vi "Configure.vi"(8 "error in (no error)":errorcluster, 9 "Record":bool, 10 "Recording Channels":refnum<k21>="All4498", 11 "AcquireTraces in":refnum<class "AcquireTraces.lvclass">) -> (0 "error out":errorcluster, 3 "AcquireTraces out":refnum<class "AcquireTraces.lvclass">)   [LabVIEW 2014, in "AcquireTraces.lvclass"]
uses:
  AcquireTraces.lvclass
  AcquireTraces.lvclass/AcquireTraces.ctl
  <vilib>/DAQmx/configure/timing.llb/DAQmx Timing (Sample Clock).vi
  <resource>/objmgr/daqmx.rc
panel:
  out "Name":refnum<k21>
  out "error out 2":errorcluster
  out "x/y":dbl
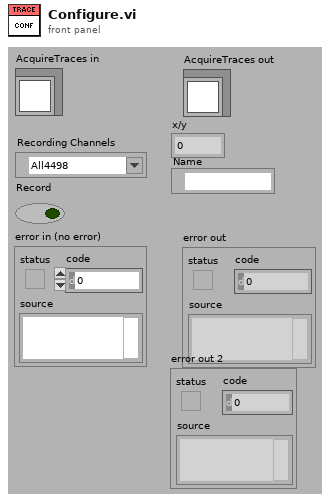
[diagram p1: front panel]
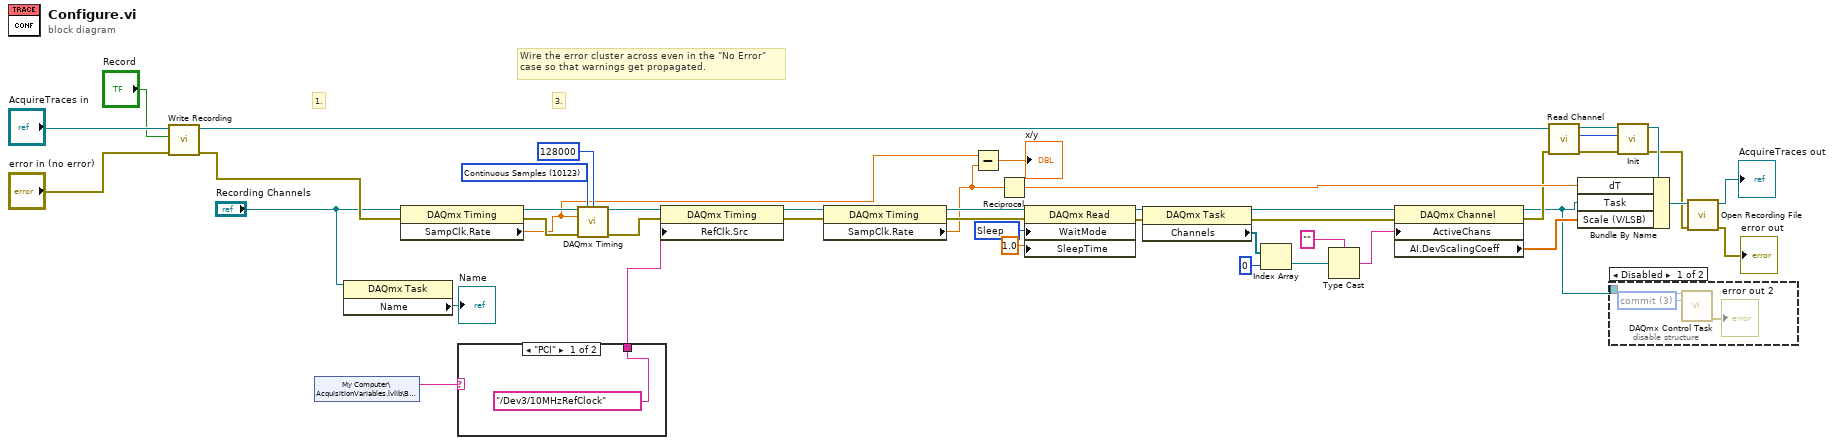
[diagram p0: block diagram]
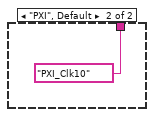
[diagram p2: hidden frame]
diagram:
  w35 = 12547 items=["Wait For Interrupt"=12523, "Poll"=12524, "Yield"=12525, "Sleep"=12547] ("WaitMode")
  w39 = 10123 items=["Finite Samples"=10178, "Continuous Samples"=10123, "Hardware Timed Single Point"=12522] ("sample mode")
  # "3."
  # "1."
  # "Wire the error cluster across even in the \"No Error\"\ncase so that warnings get propagated."
  n1 = call-dynamic "Write Recording.vi"("error in (no error)"="error in (no error)", "Recording"="Record", "AcquireTraces in"="AcquireTraces in") -> ("error out"=w9:errorcluster, "AcquireTraces out"=w6:refnum<class "AcquireTraces.lvclass">)  [unwired: 7 in]
  n2 = shared-variable "My Computer\\AcquisitionVariables.lvlib\\Bus System"() -> (w2:string)  [unwired: 1 in, 1 out]
  n3 = property class="DAQmx Task"(reference="Recording Channels") -> ("Name"=→"Name":refnum<k21>)  [unwired: 1 in, 2 out]
  n4 = property class="DAQmx Timing"(reference="Recording Channels", error in=w9) -> (reference out=w22:refnum<k21>, error out=w23:errorcluster, "SampClk.Rate"=w15:dbl)
  n5 = case shown="\"PCI\"" w2 {
    tunnel: [tag "/Dev3/10MHzRefClock" ("CI.CountEdges.Term") tag "PXI_Clk10" ("CI.CountEdges.Term")] -> w1
    frame "PCI" {
    }
    frame "PXI", Default {
    }
  }
  n6 = call-poly <vilib>:"DAQmx Timing.vi"("task/channels in"=w22, "sample mode"=w39, "samples per channel"=128000, "rate"=w15, "error in"=w23) -> ("task out"=w13:refnum<k21>, "error out"=w11:errorcluster)  [unwired: 9 in]
  n7 = property class="DAQmx Timing"(reference=w13, error in=w11, "RefClk.Src"=w1) -> (reference out=w12:refnum<k21>, error out=w10:errorcluster)
  n8 = property class="DAQmx Timing"(reference=w12, error in=w10) -> (reference out=w37:refnum<k21>, error out=w34:errorcluster, "SampClk.Rate"=w16:dbl)
  n9 = Subtract(x=w15, y=w16) -> (x-y=→"x/y":dbl)
  n10 = Reciprocal(x=w16) -> (1/x=w33:dbl)
  n11 = property class="DAQmx Read"(reference=w37, error in=w34, "WaitMode"=w35, "SleepTime"=1.0) -> (reference out=w31:refnum<k21>, error out=w30:errorcluster)
  n12 = property class="DAQmx Task"(reference=w31, error in=w30) -> (reference out=w29:refnum<k21>, error out=w28:errorcluster, "Channels"=w21:refnum<k21>[])
  n13 = Index Array(array=w21, index=0) -> (element=w26:refnum<k21>)
  n14 = Type Cast(type="", x=w26) -> (*(type *) &x=w24:string)
  n15 = property class="DAQmx Channel"(reference=w29, error in=w28, "ActiveChans"=w24) -> (reference out=w5:refnum<k21>, error out=w8:errorcluster, "AI.DevScalingCoeff"=w20:dbl[])
  n16 = call-dynamic "Read Channel.vi"("error in (no error)"=w8, "AcquistionObject in"=w6) -> ("error out"=w40:errorcluster, "Channel"=w42:i16, "AcquistionObject out"=w41:refnum<class "AcquireTraces.lvclass">)  [unwired: 7 in]
  n17 = disable-structure shown="Disabled" {
    disable-tunnel: w5 -> [w50 _]
    frame Disabled {
      w49 = 3 items=["verify"=2, "reserve"=4, "commit"=3, "unreserve"=5, "abort"=6] ("action")
      n18 = call <vilib>:"DAQmx Control Task.vi"("task/channels in"=w50, "action"=w49) -> ("error out"=→"error out 2":errorcluster)  [unwired: 12 in, 1 out]
    }
    frame Enabled {
    }
  }
  n19 = call-dynamic "Init.vi"("error in (no error)"=w40, "Channel"=w42, "AcquistionObject in"=w41) -> ("error out"=w7:errorcluster, "AcquistionObject out"=w45:refnum<class "AcquireTraces.lvclass">)  [unwired: 7 in]
  n20 = Bundle By Name(cluster=w45, "dT"=w33, "Task"=w5, "Scale (V/LSB)"=w20) -> (w32:refnum<class "AcquireTraces.lvclass">)
  n21 = call-dynamic "Open Recording File.vi"("error in (no error)"=w7, "AcquireTraces in"=w32) -> ("error out"=→"error out":errorcluster, "AcquireTraces out"=→"AcquireTraces out":refnum<class "AcquireTraces.lvclass">)  [unwired: 8 in]
